vi "Deserialize Core.vi"(8 "error in (no error)":errorcluster, 10 "Serialized Attributes":string, 11 "Serialize in":refnum<class "Display Text Msg.lvclass">) -> (0 "error out":errorcluster, 3 "Serialize out":refnum<class "Display Text Msg.lvclass">)   [LabVIEW 2020, in "Chat Window.lvlib" / "Display Text Msg.lvclass"]
uses:
  Display Text Msg.lvclass
  Display Text Msg.lvclass/Display Text Msg.ctl
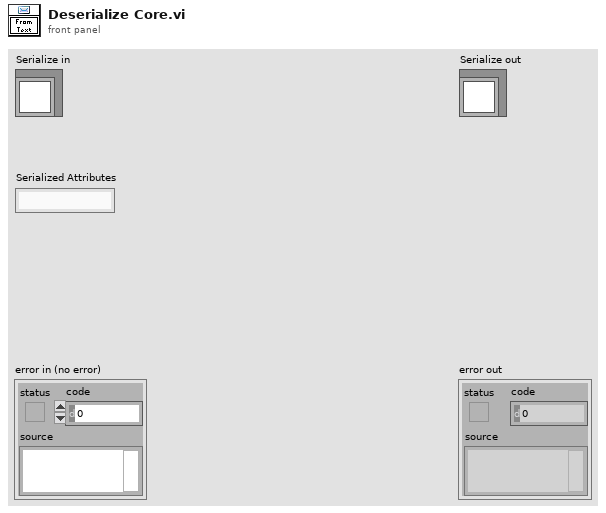
[diagram p1: front panel]
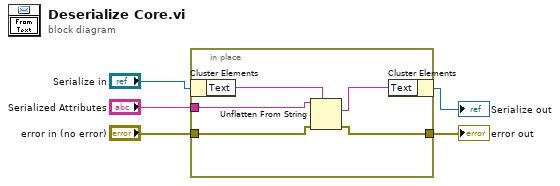
[diagram p0: block diagram]
diagram:
  n1 = in-place "In Place Element Structure" {
    in-place-border: "Serialized Attributes" -> [w10]
    in-place-border: "error in (no error)" -> [w7]
    in-place-border: [w6] -> w2
    n2 = in-place-cluster #1("Serialize in") -> ("Text"=w9:string)
    n3 = Unflatten From String(type=w9, binary string=w10, error in (no error)=w7) -> (value=w8:string, error out=w6:errorcluster)  [unwired: 2 in, 1 out]
    n4 = in-place-cluster #1("Text"=w8) -> (→"Serialize out":refnum<class "Display Text Msg.lvclass">)
  }
  "error out" <- w2
